vi "PLC_ChannelOut.vi"(3 "error in (no error)":errorcluster, 4 "Selection":T1(ring), 5 "Resistor":i32[](array[numeric]), 6 "VISA resource name":refnum<visa-resource-name>) -> (0 "error out":errorcluster)   [LabVIEW 2015]
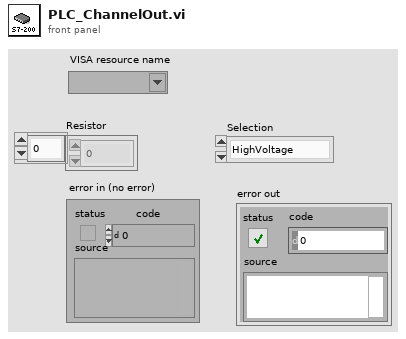
[diagram p1: front panel]
types:
  T1 = enum16{"HighVoltage", "LowVoltage", "Temperature"}
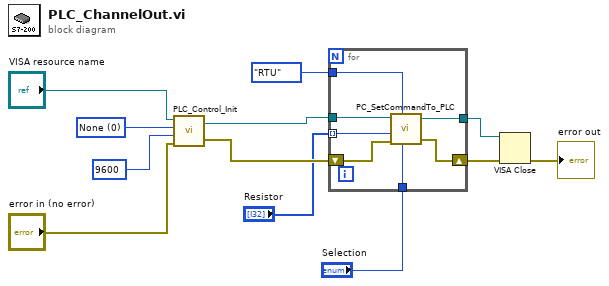
[diagram p0: block diagram]
diagram:
  w8 = u16 0 items=["None", "Odd", "Even", "Mark", "Space"] ("Parity")
  n1 = call "PLC_Control_Init.vi"("error in (no error)"="error in (no error)", "Baud Rate"=u32 9600, "Parity"=w8, "VISA resource name"="VISA resource name") -> ("error out"=w10:errorcluster, "VISA resource name out"=w2:refnum<visa-resource-name>)  [unwired: 2 in]
  n2 = for {
    tunnel: enum16{"RTU", "ASCII"}."RTU" ("Mode") -> [w15]
    tunnel: "Resistor" -> [w14] mode=indexing
    shift-right: [w18] -> w11
    shift-left: w10 -> [w17]
    tunnel: w2 -> [w16]
    tunnel: [w19] -> w12
    tunnel: "Selection" -> [w13]
    n3 = call "PC_SetCommandTo_PLC.vi"("VISA resource name"=w16, "Mode"=w15, "Resistor"=w14, "Selection"=w13, "error in (no error)"=w17) -> ("VISA resource name out"=w19:refnum<visa-resource-name>, "error out"=w18:errorcluster)  [unwired: 2 in]
  }
  n4 = VISA Close(VISA resource name=w12, error in (no error)=w11) -> (error out=→"error out":errorcluster)
